vi "LWXPS_PositionerCompensatedFastPCOCurrentStatusGet.vi"(0 "XPS Reference IN":refnum<k24>, 7 "Positioner Name":string, 11 "LabVIEW error IN":errorcluster) -> (4 "XPS Reference OUT":refnum<k24>, 6 "Returned error code":i32, 8 "Status":i32, 10 "XPS Error String":string, 15 "LabVIEW error OUT":errorcluster)   [LabVIEW 2014]
uses:
  D:/XPSQ8_LabView_Library/Development/Source/Dll/Newport.XPS.CommandInterface.dll
  Dll/Newport.XPS.CommandInterface.dll
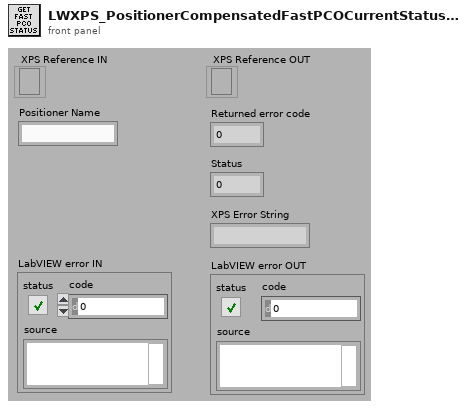
[diagram p1: front panel]
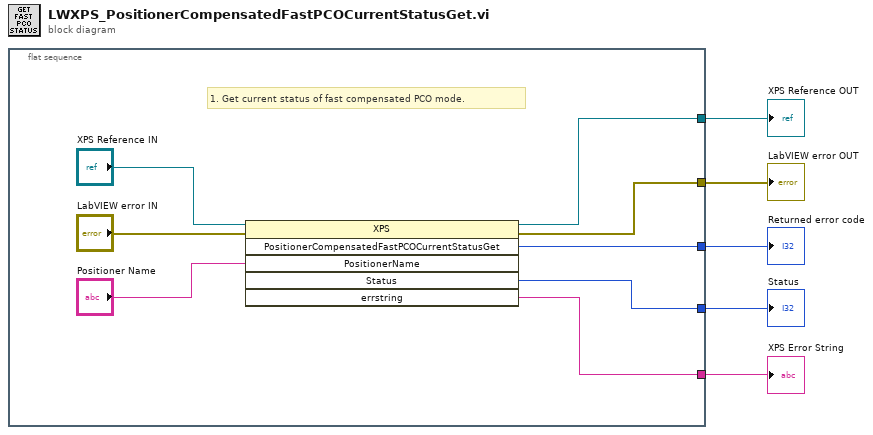
[diagram p0: block diagram]
diagram:
  n1 = flat-sequence {
    tunnel: [w6] -> w5
    tunnel: [w12] -> w4
    tunnel: [w9] -> w3
    tunnel: [w8] -> w1
    tunnel: [w7] -> w2
    frame #0 {
      # "1. Get current status of fast compensated PCO mode."
      n2 = invoke class="XPS" method="PositionerCompensatedFastPCOCurrentStatusGet"(reference="XPS Reference IN", error in="LabVIEW error IN", "PositionerName"="Positioner Name") -> (reference out=w6:refnum<k24>, error out=w12:errorcluster, "PositionerCompensatedFastPCOCurrentStatusGet"=w9:i32, "Status"=w8:i32, "errstring"=w7:string)  [unwired: 3 in, 1 out]
    }
  }
  "XPS Error String" <- w2
  "XPS Reference OUT" <- w5
  "LabVIEW error OUT" <- w4
  "Returned error code" <- w3
  "Status" <- w1
